vi "main2.vi"() -> ()   [LabVIEW 2015]
uses:
  myControl/calculationButton.ctl
  myControl/ChoseFromGraph.ctl
  myControl/Ok.ctl
  myControl/stopButton.ctl
  myControl/Events.ctl
  myControl/State.ctl
  <vilib>/Analysis/baseanly.llb/Mean (DBL).vi
  <vilib>/measure/mamon.llb/Waveform Peak Detection for 1 Chan.vi
  <vilib>/measure/NI_MAPro.lvlib
  <vilib>/Analysis/NI_AALBase.lvlib
panel:
  out "Title":string="Oscillatory Breathing Detection (beta 1.3)"
  in  "File Index:":path
  in  "Width (s):":i32
  in  "Threshold (L/min):":dbl format="%#.2g"
  in  "Low Cut-off (Hz):":dbl
  in  "OK Button":T1
  in  "ChooseFromGraph":T2
  in  "Calculate":T3
  in  "Stop Button":bool
  out "Ventilation":cluster{"Y":dbl[], "Y":dbl[]}[](graph)=[{"Y"=array[6401 elements], "Y"=array[8192 elements]}, {"Y"=[2.0, 11.0, 13.0, 16.0, 17.0, 20.0, 22.0, 24.0, 27.0, 30.0, 32.0, 36.0, 37.0, 40.0, 43.0, 45.0, 48.0, 51.0, 53.0, 55.0, 57.0, 61.0, 64.0, 66.0, 68.0, 71.0, 73.0, 75.0, 78.0, 81.0, 84.0, 86.0, 89.0, 92.0, 93.0, 96.0, 99.0, 101.0, 103.0, 107.0, 109.0, 112.0, 115.0, 118.0, 120.0, 124.0, 127.0, 129.0, 132.0, 134.0, 138.0], "Y"=[10.8, 11.5, 6.4, 8.0, 9.0, 13.8, 11.9, 14.1, 11.5, 15.7, 10.1, 14.3, 19.8, 19.2, 16.5, 21.5, 18.1, 18.9, 16.0, 17.4, 14.8, 15.3, 12.8, 11.8, 11.0, 12.4, 11.2, 12.5, 12.3, 11.5, 21.7, 21.2, 19.1, 23.7, 21.3, 20.4, 21.9, 18.3, 18.8, 17.7, 12.9, 12.6, 11.4, 9.9, 11.1, 12.3, 15.6, 14.5, 16.0, 14.2, 16.4]}]
  out "Duration (s)":dbl[](array[numeric]) format="%#.2g"
  out "Amplitude (L/min)":dbl[](array[numeric]) format="%#.2g"
  out "Mean Area Ratio":dbl format="%#.2g"
  out "Mean Area":dbl format="%#.2f"
  out "iValesLocation(samples)":dbl[](array[numeric])=[127.0, 3160.0, 5625.0] format="%#.2g"
  out "Cycle Number":i32
  out "EOB Ratio":dbl format="%#.2g"
  out "Freq. (1/min)":dbl format="%#.2g"
  out "Ampl. (L/min)":dbl format="%#.2g"
  out "DataArray":T4
  out "State Bar":string="Set the Run-Time settings and press Calculate Button "
  # "Preliminary Setting:"
  # "Run-Time Setting:"
  # "Detected cycles:"
  # "Average values:"
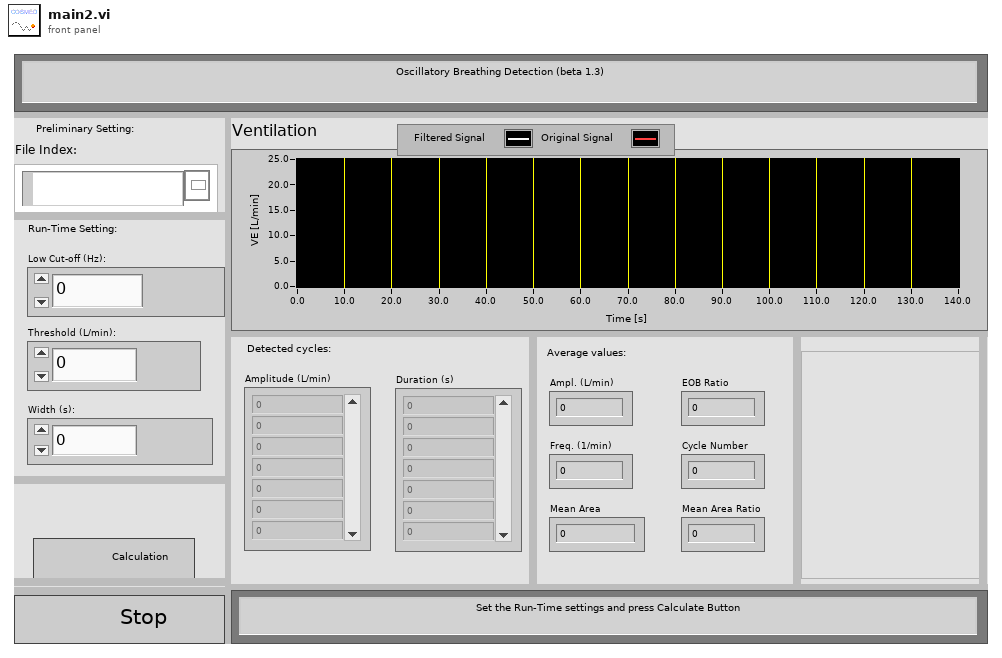
[diagram p1: front panel]
types:
  T1 = typedef "Ok.ctl" = bool
  T2 = typedef "ChoseFromGraph.ctl" = bool
  T3 = typedef "calculationButton.ctl" = bool
  T4 = cluster{"VE_E":dbl[], "time_E":dbl[], "VE_B":dbl[], "time_B":dbl[], "VE_E_noInter":dbl[], "time_E_noInter":dbl[], "VE_B_noInter":dbl[], "time_B_noInter":dbl[], "filteredSignal":dbl[], "iPeaksLocation":dbl[], "peaksAmplitude":dbl[], "valesAmplitude":dbl[], "iValesLocation":dbl[], "#_peaksFound":i32, "iPeakLocation_User":dbl[], "peakAmplitude_User":dbl[]}
  T5 = typedef "stopButton.ctl" = bool
  T6 = typedef "State.ctl" = enum16{"Inizializing", "UpLoad&ControlFile", "CalculationDefaultWidth", "WaitEvent", "Filter", "ChooseFromGraph", "FindPeaks", "FindVales", "TestOscillation", "CalculationOscillation", "Stop"}
  T7 = typedef "Events.ctl" = enum16{"WaitEvent", "ChoseFile", "Calculate", "ChoseFromGraoph", "Stop"}
  T8 = cluster{"time_E_noInter":dbl[], "VE_E_noInter":dbl[]}
  T9 = cluster{"time_E_noInter":dbl[], "VE_E_noInter":dbl[]}[]
  T10 = typedef "LVPoint32TypeDef.ctl" = cluster{"Horizontal":i32, "Vertical":i32}
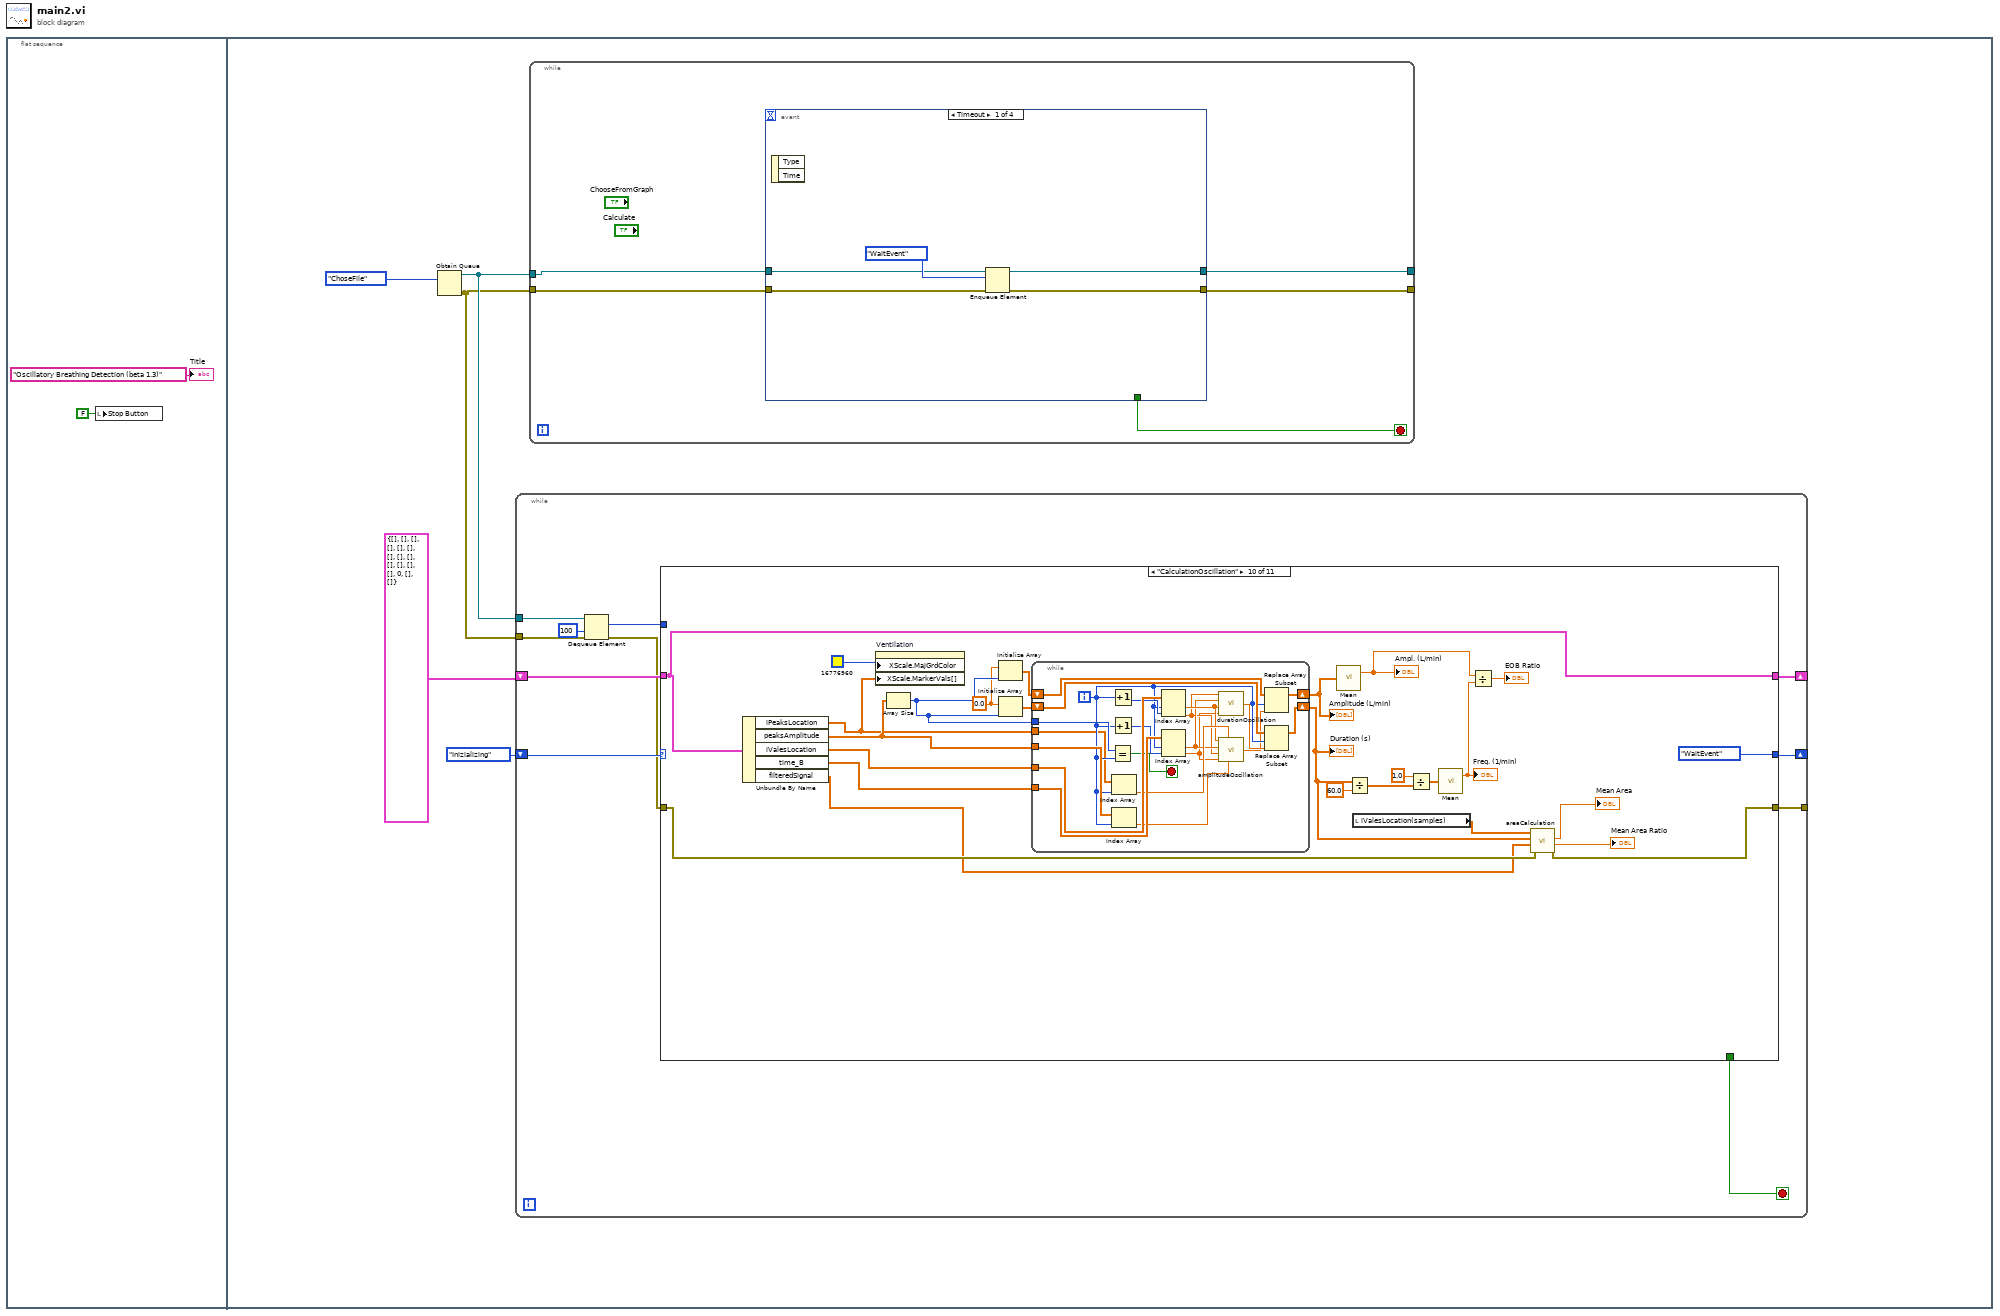
[diagram p0: block diagram]
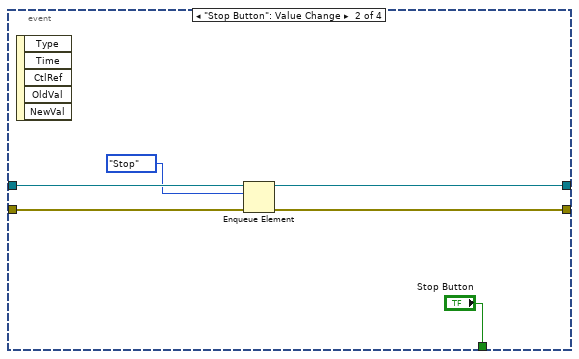
[diagram p2: hidden frame]
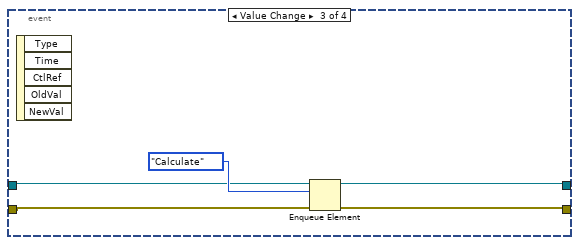
[diagram p3: hidden frame]
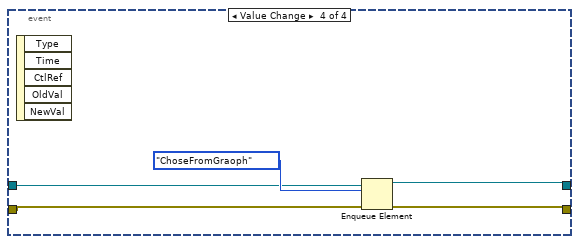
[diagram p4: hidden frame]
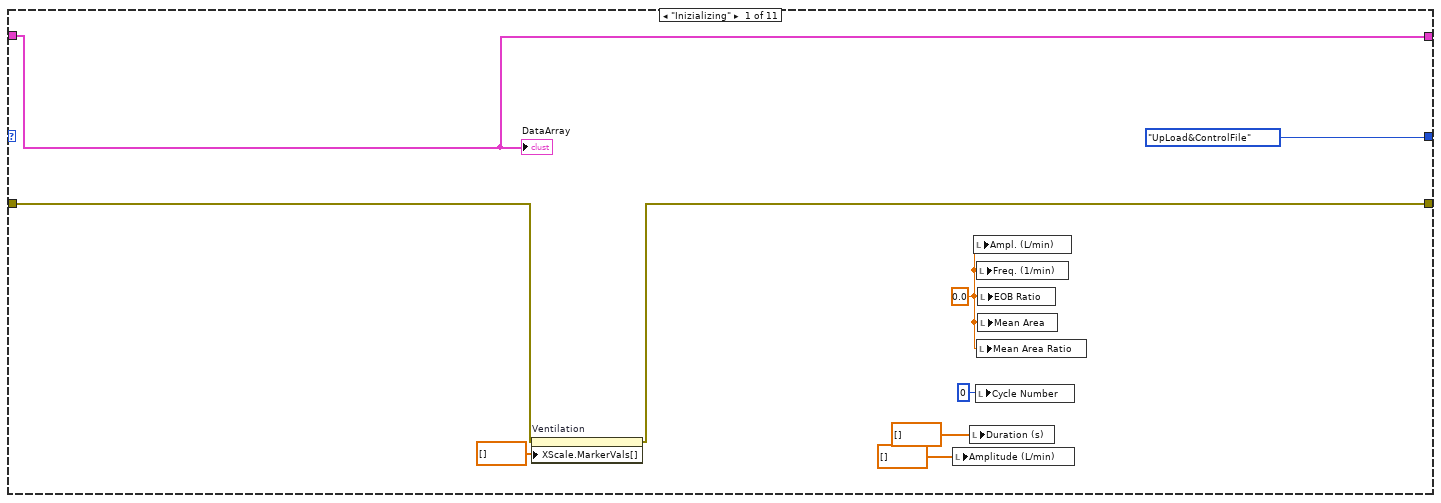
[diagram p5: hidden frame]
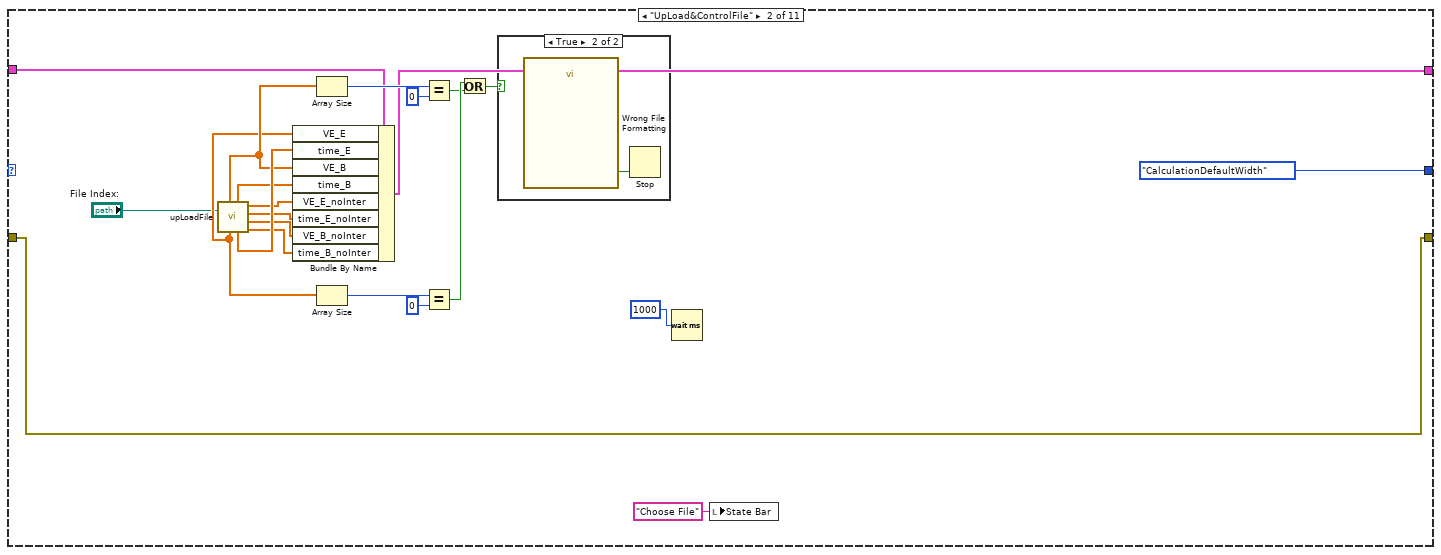
[diagram p6: hidden frame]
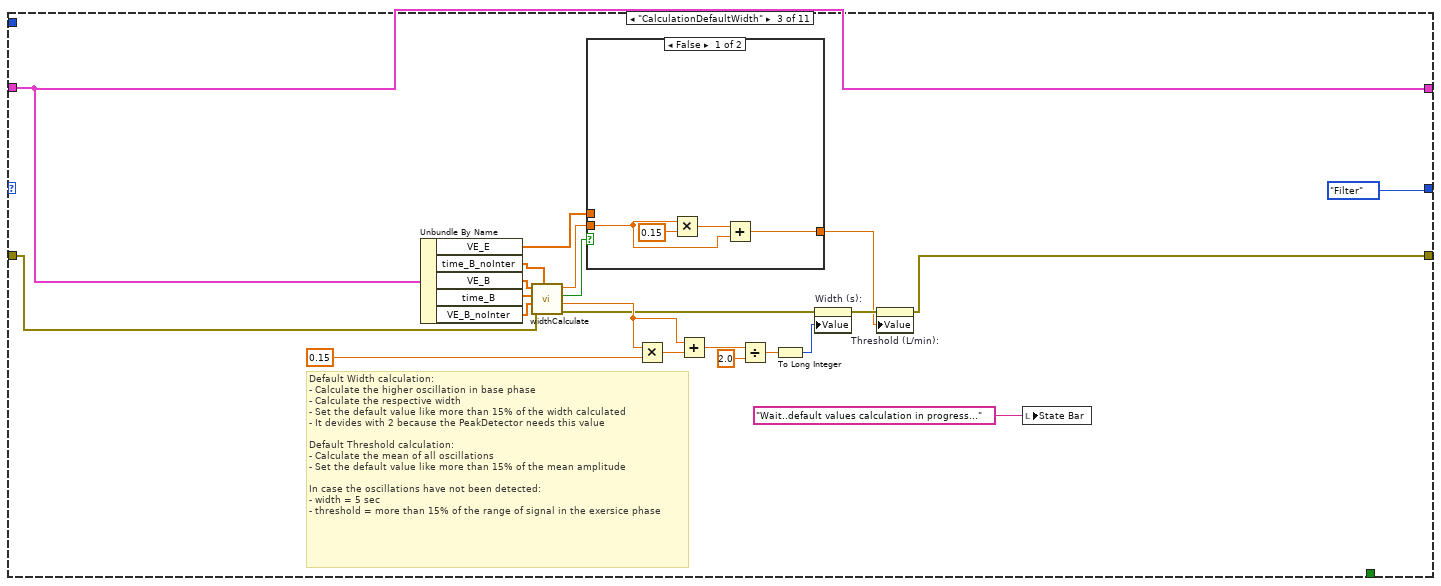
[diagram p8: hidden frame]
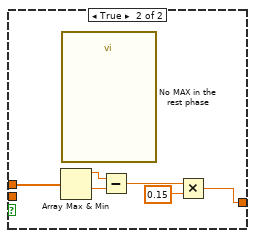
[diagram p9: hidden frame]
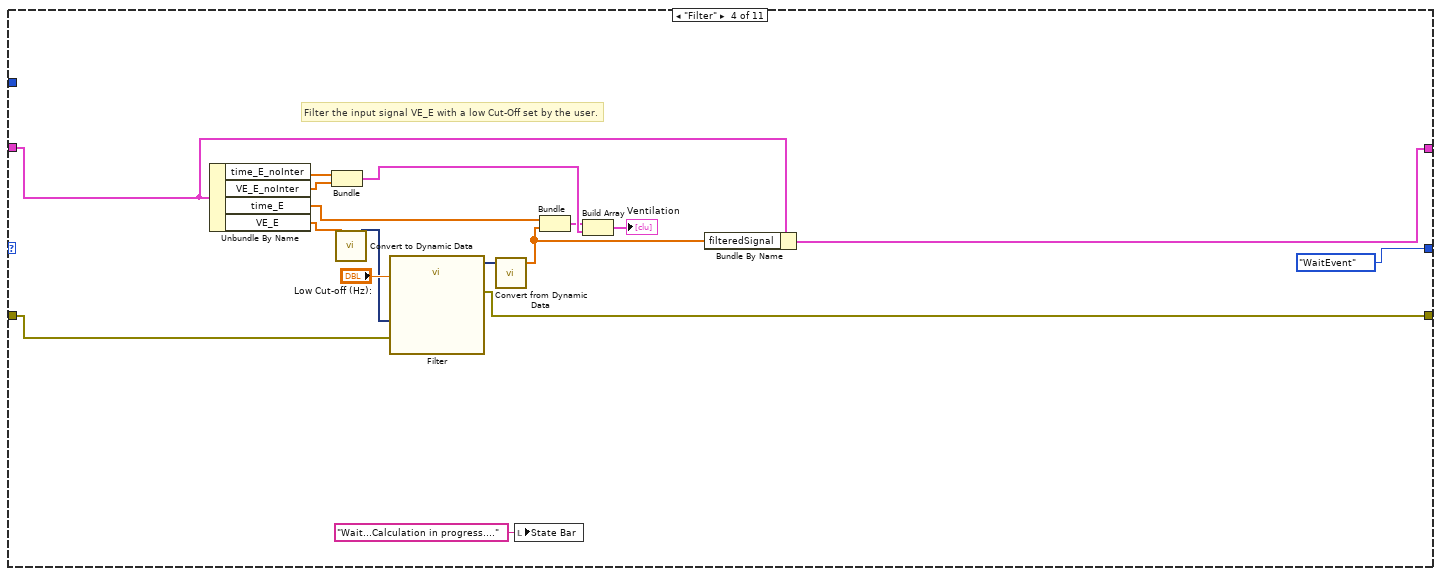
[diagram p10: hidden frame]
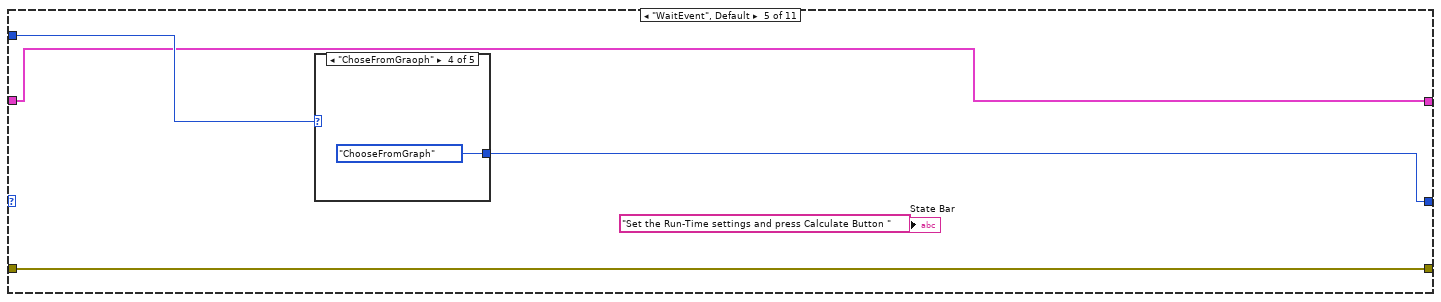
[diagram p11: hidden frame]
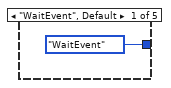
[diagram p12: hidden frame]
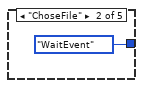
[diagram p13: hidden frame]
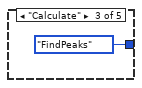
[diagram p14: hidden frame]
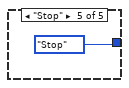
[diagram p15: hidden frame]
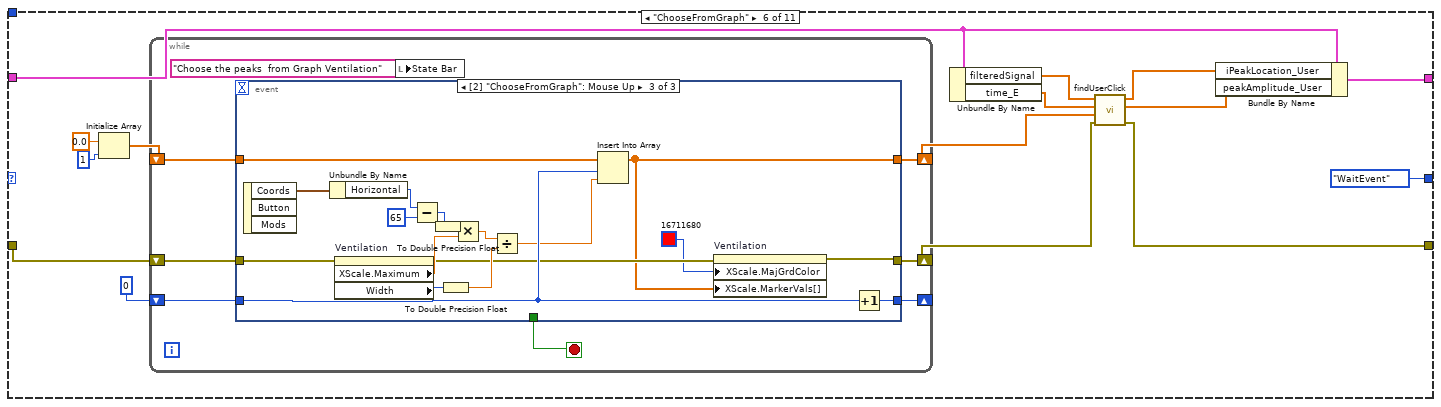
[diagram p16: hidden frame]
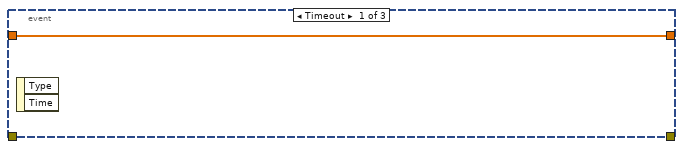
[diagram p17: hidden frame]
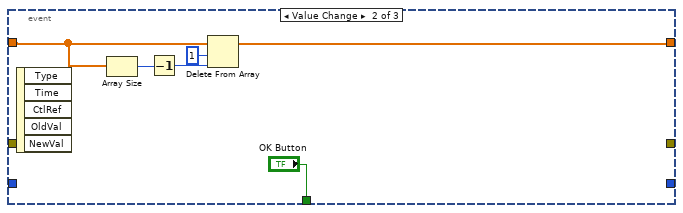
[diagram p18: hidden frame]
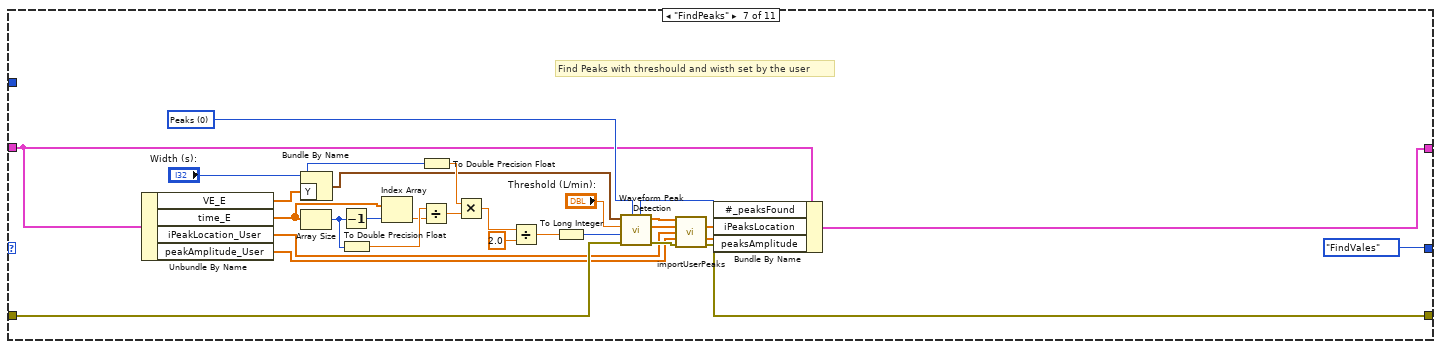
[diagram p19: hidden frame]
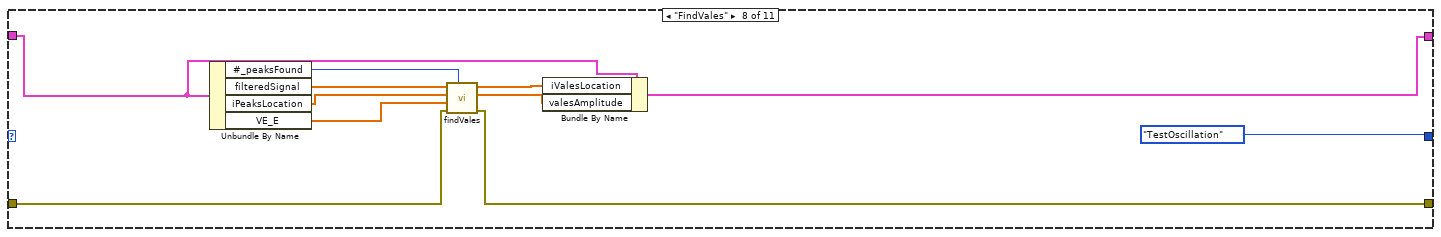
[diagram p20: hidden frame]
diagram:
  n1 = flat-sequence {
    frame #0 {
      n2 = local write "Stop Button"(T5 FALSE ("Stop Button")) -> ()
      "Title" <- "Oscillatory Breathing Detection (beta 1.3)" ("String")
    }
    frame #1 {
      n3 = Obtain Queue(element data type=Events."ChoseFile" ("Events")) -> (queue out=w7:refnum<queue>, error out=w6:errorcluster)  [unwired: 4 in, 1 out]
      n4 = while {
        shift-right: [w43] -> _
        shift-left: State."Inizializing" ("States") -> [w44]
        tunnel: w7 -> [w42]
        tunnel: w6 -> [w41]
        shift-right: [w39] -> _
        shift-left: T4 {"VE_E"=[], "time_E"=[], "VE_B"=[], "time_B"=[], "VE_E_noInter"=[], "time_E_noInter"=[], "VE_B_noInter"=[], "time_B_noInter"=[], "filteredSignal"=[], "iPeaksLocation"=[], "peaksAmplitude"=[], "valesAmplitude"=[], "iValesLocation"=[], "#_peaksFound"=0, "iPeakLocation_User"=[], "peakAmplitude_User"=[]} ("DataArray 2") -> [w38]
        tunnel: [w36] -> _
        stop <- w34 stop-if-true
        n5 = Dequeue Element(queue=w42, timeout in ms (-1)=100, error in (no error)=w41) -> (element=w35:T7, error out=w37:errorcluster)  [unwired: 2 out]
        n6 = case shown="\"CalculationOscillation\"" w44 {
          tunnel: [State."UpLoad&ControlFile" ("States") State."CalculationDefaultWidth" ("States") State."Filter" ("States") State."WaitEvent" ("States") w129 State."WaitEvent" ("States") State."FindVales" ("States") State."TestOscillation" ("States") State."CalculationOscillation" ("States") State."WaitEvent" ("States") State."WaitEvent" ("States")] -> w43
          tunnel: w38 -> [w52 w58 w83 w113 w128 w143 w196 w217 w238 w284 w324]
          tunnel: [w52 w56 w83 w112 w128 w144 w195 w214 w237 w284 w324] -> w39
          tunnel: w37 -> [w50 w54 w85 w115 w127 w149 w194 w223 w250 w280 w321]
          tunnel: [w49 w54 w80 w114 w127 w141 w190 w222 w240 w279 w321] -> w36
          tunnel: w35 -> [_ _ _ _ w130 _ _ _ _ _ _]
          tunnel: [_ _ _ _ _ _ _ _ _ _ TRUE] -> w34
          frame "Inizializing" {
            w45 = 0.0 ("Ampl. (L/min)")
            n7 = property on="Ventilation" class="XYGraph (strict)"(error in=w50, "XScale.MarkerVals[]"=dbl[] [] ("X Scale.Marker Values[]")) -> (error out=w49:errorcluster)  [unwired: 1 in, 1 out]
            n8 = local write "Amplitude (L/min)"(dbl[] [] ("Amplitude (L/min)")) -> ()
            n9 = local write "Duration (s)"(dbl[] [] ("Duration (s)")) -> ()
            n10 = local write "Ampl. (L/min)"(w45) -> ()
            n11 = local write "Cycle Number"(0 ("Cycle Number")) -> ()
            n12 = local write "Freq. (1/min)"(w45) -> ()
            n13 = local write "Mean Area Ratio"(w45) -> ()
            n14 = local write "EOB Ratio"(w45) -> ()
            n15 = local write "Mean Area"(w45) -> ()
            "DataArray" <- w52
          }
          frame "UpLoad&ControlFile" {
            n16 = call "upLoadFile.vi"("file path (dialog if empty)"="File Index:") -> ("time_B_noInter"=w60:dbl[], "VE_B_noInter"=w61:dbl[], "time_E_noInter"=w62:dbl[], "VE_E_noInter"=w63:dbl[], "time_E"=w66:dbl[], "time_B"=w64:dbl[], "VE_E"=w59:dbl[], "VE_B"=w65:dbl[])  [unwired: 3 in]
            n17 = Bundle By Name(cluster=w58, "VE_E"=w59, "time_E"=w66, "VE_B"=w65, "time_B"=w64, "VE_E_noInter"=w63, "time_E_noInter"=w62, "VE_B_noInter"=w61, "time_B_noInter"=w60) -> (w56:T4)
            n18 = Array Size(array=w65) -> (size(s)=w69:i32)
            n19 = Array Size(array=w59) -> (size(s)=w73:i32)
            n20 = Equal?(x=w69, y=0) -> (x = y?=w67:bool)
            n21 = Equal?(x=w73, y=0) -> (x = y?=w71:bool)
            n22 = Or(x=w71, y=w67) -> (x .or. y?=w70:bool)
            n23 = case shown="True" w70 {
              frame False {
              }
              frame True {
                n24 = call "Wrong File Formatting"() -> ("OK"=w76:bool)  [unwired: 10 in, 1 out]
                n25 = Stop(stop? (T)=w76) -> ()
              }
            }
            n26 = Wait (ms)(milliseconds to wait=u32 1000) -> ()  [unwired: 1 out]
            n27 = local write "State Bar"("Choose File" ("State Bar")) -> ()
          }
          frame "CalculationDefaultWidth" {
            # "Default Width calculation:\n- Calculate the higher oscillation in base phase\n- Calculate the respective width\n- Set the default value like more than 15% of the width calculated\n- It devides with 2 because the PeakDetector needs this value\n\nDefault Threshold calculation:\n- Calculate the mean of all oscillations\n- Set the default value like more than 15% of the mean amplitude\n\nIn case the oscillations have not been detected:\n- width = 5 sec\n- threshold = more than 15% of the range of signal in the exersice phase"
            n28 = Unbundle By Name(w83) -> ("VE_E"=w77:dbl[], "time_B_noInter"=w86:dbl[], "VE_B"=w89:dbl[], "time_B"=w88:dbl[], "VE_B_noInter"=w87:dbl[])
            n29 = call "widthCalculate.vi"("time_B_noInter"=w86, "Error In"=w85, "VE_B_noInter"=w87, "time_B"=w88, "VE_B"=w89) -> ("Error Out"=w82:errorcluster, "maxWidth"=w93:dbl, "noMin"=w98:bool, "Ampl. (L/min)"=w79:dbl)
            n30 = case shown="False" w98 {
              tunnel: w79 -> [w100 _]
              tunnel: [w99 w103] -> w78
              tunnel: w77 -> [_ w108]
              frame False {
                n31 = Multiply(x=w100, y=0.15) -> (x*y=w101:dbl)
                n32 = Add(x=w101, y=w100) -> (x+y=w99:dbl)
              }
              frame True {
                n33 = Array Max & Min(array=w108) -> (max value=w107:dbl, min value=w106:dbl)  [unwired: 2 out]
                n34 = call "No MAX in the rest phase"() -> ()  [unwired: 10 in, 2 out]
                n35 = Subtract(x=w107, y=w106) -> (x-y=w105:dbl)
                n36 = Multiply(x=w105, y=0.15) -> (x*y=w103:dbl)
              }
            }
            n37 = Multiply(x=w93, y=0.15) -> (x*y=w92:dbl)
            n38 = Add(x=w93, y=w92) -> (x+y=w91:dbl)
            n39 = Divide(x=w91, y=2.0) -> (x/y=w95:dbl)
            n40 = To Long Integer(number=w95) -> (32bit integer=w90:i32)
            n41 = property on="Width (s):" class="DigNum (strict)"(error in=w82, "Value"=w90) -> (error out=w81:errorcluster)  [unwired: 1 in, 1 out]
            n42 = property on="Threshold (L/min):" class="DigNum (strict)"(error in=w81, "Value"=w78) -> (error out=w80:errorcluster)  [unwired: 1 in, 1 out]
            n43 = local write "State Bar"("Wait..default values calculation in progress..." ("State Bar")) -> ()
          }
          frame "Filter" {
            # "Filter the input signal VE_E with a low Cut-Off set by the user."
            n44 = Unbundle By Name(w113) -> ("time_E_noInter"=w119:dbl[], "VE_E_noInter"=w118:dbl[], "time_E"=w117:dbl[], "VE_E"=w116:dbl[])
            n45 = Bundle("time_E_noInter"=w119, "VE_E_noInter"=w118) -> (w125:T8)  [unwired: 1 in]
            n46 = call "Convert to Dynamic Data"("Array"=w116) -> ("Dynamic Data Type"=w121:dynamicdata)  [unwired: 3 in]
            n47 = call "Filter"("error in (no error)"=w115, "Lower Cut-Off"="Low Cut-off (Hz):", "Signal"=w121) -> ("error out"=w114:errorcluster, "Filtered Signal"=w122:dynamicdata)  [unwired: 7 in]
            n48 = call "Convert from Dynamic Data"("Dynamic Data Type"=w122) -> ("Array"=w109:dbl[])  [unwired: 3 in]
            n49 = local write "State Bar"("Wait...Calculation in progress...." ("String 2")) -> ()
            n50 = Bundle("time_E"=w117, "Array"=w109) -> (w123:cluster{"time_E":dbl[], "Array":dbl[]})  [unwired: 1 in]
            n51 = Build Array(w123, w125) -> (→"Ventilation":T9)
            n52 = Bundle By Name(cluster=w113, "filteredSignal"=w109) -> (w112:T4)
          }
          frame "WaitEvent", Default {
            n53 = case shown="\"ChoseFromGraoph\"" w130 {
              tunnel: [State."WaitEvent" ("States") State."WaitEvent" ("States") State."FindPeaks" ("States") State."ChooseFromGraph" ("States") State."Stop" ("States")] -> w129
              frame "WaitEvent", Default {
              }
              frame "ChoseFile" {
              }
              frame "Calculate" {
              }
              frame "ChoseFromGraoph" {
              }
              frame "Stop" {
              }
            }
            "State Bar" <- "Set the Run-Time settings and press Calculate Button " ("State Bar")
          }
          frame "ChooseFromGraph" {
            n54 = Initialize Array(0.0 ("element"), 1 ("dimension size")) -> (w145:dbl[])
            n55 = while {
              shift-right: [w152] -> w142
              shift-left: w149 -> [w158]
              shift-right: [w154] -> w140
              shift-left: w145 -> [w157]
              shift-right: [w155] -> _
              shift-left: 0 ("element") -> [w156]
              stop <- w151 stop-if-true
              n56 = event shown="[2] \"ChooseFromGraph\": Mouse Up" {
                selector: _ -> [_ _ _]
                dyn-events: _ -> [_ _ _]
                timeout: _ -> [_ _ _]
                tunnel: w158 -> [_ _ w183]
                tunnel: w157 -> [w159 w164 w172]
                tunnel: w156 -> [_ _ w171]
                tunnel: [_ _ w173] -> w155
                tunnel: [w159 w165 w167] -> w154
                tunnel: [_ _ w168] -> w152
                tunnel: [_ "OK Button" _] -> w151
                event Timeout {
                  n57 = event-data() -> ()  [unwired: 1 in, 2 out]
                }
                event Value Change {
                  n58 = event-data() -> ()  [unwired: 1 in, 5 out]
                  n59 = Array Size(array=w164) -> (size(s)=w163:i32)
                  n60 = Decrement(x=w163) -> (x-1=w161:i32)
                  n61 = Delete From Array(array=w164, length=1, index=w161) -> (array with subset deleted=w165:dbl[])  [unwired: 1 out]
                }
                event Mouse Up {
                  n62 = event-data() -> ("Coords"=w182:T10)  [unwired: 1 in, 2 out]
                  n63 = Unbundle By Name(w182) -> ("Horizontal"=w181:i32)
                  n64 = property on="Ventilation" class="XYGraph (strict)"(error in=w183) -> (error out=w169:errorcluster, "XScale.Maximum"=w179:dbl, "Width"=w175:u32)  [unwired: 1 in, 1 out]
                  n65 = Subtract(x=w181, y=65) -> (x-y=w178:i32)
                  n66 = To Double Precision Float(number=w178) -> (double precision float=w177:dbl)
                  n67 = To Double Precision Float(number=w175) -> (double precision float=w174:dbl)
                  n68 = Multiply(x=w177, y=w179) -> (x*y=w176:dbl)
                  n69 = Divide(x=w176, y=w174) -> (x/y=w170:dbl)
                  n70 = Insert Into Array(array=w172, index=w171, new element=w170) -> (w167:dbl[])
                  n71 = property on="Ventilation" class="XYGraph (strict)"(error in=w169, "XScale.MajGrdColor"=u32 16711680 ("Color Box"), "XScale.MarkerVals[]"=w167) -> (error out=w168:errorcluster)  [unwired: 1 in, 1 out]
                  n72 = Increment(x=w171) -> (x+1=w173:i32)
                }
              }
              n73 = local write "State Bar"("Choose the peaks  from Graph Ventilation" ("State Bar")) -> ()
            }
            n74 = Unbundle By Name(w143) -> ("filteredSignal"=w138:dbl[], "time_E"=w139:dbl[])
            n75 = call "findUserClick.vi"("Error In"=w142, "clickLocation"=w140, "time_E"=w139, "VE_amplitude"=w138) -> ("Error Out"=w141:errorcluster, "amplitudePeaks"=w136:dbl[], "iPeaksLocation"=w137:dbl[])  [unwired: 5 in]
            n76 = Bundle By Name(cluster=w143, "iPeakLocation_User"=w137, "peakAmplitude_User"=w136) -> (w144:T4)
          }
          frame "FindPeaks" {
            w200 = u16 0 items=["Peaks", "Valleys"] ("peaks/valleys")
            # "Find Peaks with threshould and wisth set by the user"
            n77 = Unbundle By Name(w196) -> ("VE_E"=w197:dbl[], "time_E"=w198:dbl[], "iPeakLocation_User"=w185:dbl[], "peakAmplitude_User"=w184:dbl[])
            n78 = Bundle By Name("Y"=w197) -> (w201:waveform(dbl))  [unwired: 1 in]
            n79 = Array Size(array=w198) -> (size(s)=w209:i32)
            n80 = Decrement(x=w209) -> (x-1=w211:i32)
            n81 = To Double Precision Float(number=w209) -> (double precision float=w210:dbl)
            n82 = Index Array(array=w198, index=w211) -> (element=w199:dbl)
            n83 = Divide(x=w210, y=w199) -> (x/y=w212:dbl)
            n84 = To Double Precision Float(number="Width (s):") -> (double precision float=w204:dbl)
            n85 = Multiply(x=w204, y=w212) -> (x*y=w206:dbl)
            n86 = Divide(x=w206, y=2.0) -> (x/y=w208:dbl)
            n87 = To Long Integer(number=w208) -> (32bit integer=w205:i32)
            n88 = call-poly <vilib>:"Waveform Peak Detection.vi"("peaks/valleys"=w200, "error in"=w194, "width"=w205, "threshold"="Threshold (L/min):", "Signal In"=w201) -> ("error out"=w191:errorcluster, "Amplitudes"=w187:dbl[], "Locations"=w186:dbl[], "# found"=w193:i32)  [unwired: 2 in, 1 out]
            n89 = call "importUserPeaks.vi"("iPeak_Location"=w186, "amplitudePeaks"=w187, "iPeak_LocationUSER"=w185, "amplitudePeaksUSER"=w184, "Error In"=w191) -> ("iPeak_LocationFinal"=w189:dbl[], "amplitudePeaksFinal"=w188:dbl[], "Error Out"=w190:errorcluster)  [unwired: 8 in]
            n90 = Bundle By Name(cluster=w196, "#_peaksFound"=w193, "iPeaksLocation"=w189, "peaksAmplitude"=w188) -> (w195:T4)
          }
          frame "FindVales" {
            n91 = Unbundle By Name(w217) -> ("#_peaksFound"=w221:i32, "filteredSignal"=w220:dbl[], "iPeaksLocation"=w219:dbl[], "VE_E"=w218:dbl[])
            n92 = call "findVales.vi"("#_foundPeaks"=w221, "Error In"=w223, "VE_E"=w218, "iPeaksLocation"=w219, "filteredSignal"=w220) -> ("Error Out"=w222:errorcluster, "valesAmplitude"=w215:dbl[], "iValesLocation"=w216:dbl[])  [unwired: 4 in]
            n93 = Bundle By Name(cluster=w217, "iValesLocation"=w216, "valesAmplitude"=w215) -> (w214:T4)
          }
          frame "TestOscillation" {
            w245 = 0.0 ("element")
            n94 = local read "Threshold (L/min):"() -> (w251:dbl)
            n95 = Unbundle By Name(w238) -> ("#_peaksFound"=w254:i32, "valesAmplitude"=w253:dbl[], "peaksAmplitude"=w252:dbl[])
            n96 = Unbundle By Name(w238) -> ("time_E"=w239:dbl[], "filteredSignal"=w231:dbl[], "peaksAmplitude"=w230:dbl[], "iValesLocation"=w225:dbl[], "iPeaksLocation"=w229:dbl[], "valesAmplitude"=w228:dbl[])
            n97 = call "verifyThreshold.vi"("#Peaks"=w254, "valesAmplitude"=w253, "peaksAmplitude"=w252, "Error In"=w250, "threshold"=w251) -> ("passThreshold"=w249:i32[], "Error Out"=w248:errorcluster)
            n98 = call "testMaxMin.vi"("valesAmplitude in"=w228, "peaksAmplitude in"=w230, "Error In"=w248, "iPeaksLocation in"=w229, "iValesLocation in"=w225, "passThreshold"=w249) -> ("Error Out"=w242:errorcluster, "iValesLocation out"=w224:dbl[], "valesAmplitude out"=w233:dbl[])  [unwired: 2 out]
            "iValesLocation(samples)" <- w224
            n99 = Array Size(array=w224) -> (size(s)=w227:i32)
            n100 = call "iToTime.vi"("Error In"=w242, "time"=w239, "iArray"=w224) -> ("Error Out"=w241:errorcluster, "timeArray"=w234:dbl[])
            n101 = Decrement(x=w227) -> (x-1=w226:i32)
            "Cycle Number" <- w226
            n102 = Initialize Array(w245, w226) -> (w244:dbl[])
            n103 = Initialize Array(w245, w226) -> (w246:dbl[])
            n104 = while {
              tunnel: w224 -> [w273]
              tunnel: w227 -> [w272]
              tunnel: w231 -> [w269]
              shift-right: [w255] -> _
              shift-left: 0 -> [w256]
              shift-right: [w266] -> w235
              shift-left: w246 -> [w267]
              shift-right: [w264] -> w243
              shift-left: w244 -> [w265]
              i -> [w263]
              stop <- w271 stop-if-true
              n105 = Increment(x=w263) -> (x+1=w259:i32)
              n106 = Equal?(x=w272, y=w263) -> (x = y?=w271:bool)
              n107 = Index Array(array=w273, index=w259) -> (element=w270:dbl)
              n108 = To Long Integer(number=w270) -> (32bit integer=w255:i32)
              n109 = Subtract(x=w255, y=w256) -> (x-y=w257:i32)
              n110 = Array Subset(array=w269, index=w256, length=w257) -> (w268:dbl[])
              n111 = Array Max & Min(array=w268) -> (max value=w261:dbl, max index (indices)=w262:i32)  [unwired: 2 out]
              n112 = Add(x=w262, y=w256) -> (x+y=w258:i32)
              n113 = Replace Array Subset(array=w267, new element=w261, index=w263) -> (w266:dbl[])
              n114 = To Double Precision Float(number=w258) -> (double precision float=w260:dbl)
              n115 = Replace Array Subset(array=w265, new element=w260, index=w263) -> (w264:dbl[])
            }
            n116 = call "iToTime.vi"("Error In"=w241, "time"=w239, "iArray"=w243) -> ("Error Out"=w240:errorcluster, "timeArray"=w236:dbl[])
            n117 = Bundle By Name(cluster=w238, "valesAmplitude"=w233, "iPeaksLocation"=w236, "peaksAmplitude"=w235, "iValesLocation"=w234) -> (w237:T4)
          }
          frame "CalculationOscillation" {
            w288 = 0.0 ("element")
            n118 = Unbundle By Name(w284) -> ("iPeaksLocation"=w282:dbl[], "peaksAmplitude"=w287:dbl[], "iValesLocation"=w286:dbl[], "time_B"=w285:dbl[], "filteredSignal"=w276:dbl[])
            n119 = property on="Ventilation" class="XYGraph (strict)"("XScale.MajGrdColor"=u32 16776960 ("Color Box"), "XScale.MarkerVals[]"=w282) -> ()  [unwired: 2 in, 2 out]
            n120 = Array Size(array=w287) -> (size(s)=w299:i32)
            n121 = Initialize Array(w288, w299) -> (w289:dbl[])
            n122 = Initialize Array(w288, w299) -> (w290:dbl[])
            n123 = while {
              tunnel: w287 -> [w320]
              tunnel: w282 -> [w300]
              tunnel: w285 -> [w319]
              tunnel: w286 -> [w318]
              tunnel: w299 -> [w317]
              shift-right: [w310] -> w277
              shift-left: w290 -> [w311]
              shift-right: [w312] -> w291
              shift-left: w289 -> [w313]
              i -> [w309]
              stop <- w316 stop-if-true
              n124 = Equal?(x=w317, y=w309) -> (x = y?=w316:bool)
              n125 = Increment(x=w309) -> (x+1=w314:i32)
              n126 = Increment(x=w309) -> (x+1=w315:i32)
              n127 = Index Array(array=w300, index=w309) -> (element=w307:dbl)
              n128 = Index Array(array=w320, index=w309) -> (element=w306:dbl)
              n129 = Index Array(array=w318, index #1=w309, index #2=w314) -> (element #1=w305:dbl, element #2=w303:dbl)
              n130 = Index Array(array=w319, index #1=w309, index #2=w315) -> (element #1=w304:dbl, element #2=w302:dbl)
              n131 = call "durationOscillation.vi"("valesAmplitude2"=w302, "timeValesLocation1"=w305, "valesAmplitude1"=w304, "timeValesLocation2"=w303) -> ("durationOscilation"=w308:dbl)
              n132 = call "amplitudeOscillation.vi"("y0"=w306, "x0"=w307, "y2"=w302, "x2"=w303, "y1"=w304, "x1"=w305) -> ("amplitudeOscillation"=w301:dbl)
              n133 = Replace Array Subset(array=w313, new element=w301, index=w309) -> (w312:dbl[])
              n134 = Replace Array Subset(array=w311, new element=w308, index=w309) -> (w310:dbl[])
            }
            "Duration (s)" <- w277
            "Amplitude (L/min)" <- w291
            n135 = call-poly <vilib>:"Mean.vi"("X"=w291) -> ("mean"=w295:dbl)  [unwired: 1 out]
            "Ampl. (L/min)" <- w295
            n136 = Divide(x=w277, y=60.0) -> (x/y=w293:dbl[])
            n137 = local read "iValesLocation(samples)"() -> (w278:dbl[])
            n138 = Divide(x=1.0, y=w293) -> (x/y=w297:dbl[])
            n139 = call-poly <vilib>:"Mean.vi"("X"=w297) -> ("mean"=w298:dbl)  [unwired: 1 out]
            "Freq. (1/min)" <- w298
            n140 = Divide(x=w295, y=w298) -> (x/y=→"EOB Ratio":dbl)
            n141 = call "areaCalculation.vi"("error in (no error)"=w280, "filteredSignal"=w276, "Duration"=w277, "iValesLocation(Samples)"=w278) -> ("error out"=w279:errorcluster, "meanArea/numOsci"=→"Mean Area Ratio":dbl, "meanArea"=→"Mean Area":dbl)  [unwired: 5 in]
          }
          frame "Stop" {
          }
        }
      }
      n142 = while {
        tunnel: w7 -> [w12]
        tunnel: w6 -> [w11]
        tunnel: [w10] -> _
        tunnel: [w9] -> _
        stop <- w8 stop-if-true
        n143 = event shown="[0] Timeout" {
          selector: _ -> [_ _ _ _]
          dyn-events: _ -> [_ _ _ _]
          timeout: _ -> [_ _ _ _]
          tunnel: w12 -> [w16 w23 w27 w32]
          tunnel: w11 -> [w15 w22 w26 w31]
          tunnel: [w14 w21 w25 w30] -> w10
          tunnel: [w13 w20 w24 w29] -> w9
          tunnel: [_ "Stop Button" _ _] -> w8
          event Timeout {
            n144 = event-data() -> ()  [unwired: 1 in, 2 out]
            n145 = Enqueue Element(queue=w16, element=Events."WaitEvent" ("Events"), error in (no error)=w15) -> (queue out=w14:refnum<queue>, error out=w13:errorcluster)  [unwired: 1 in, 1 out]
          }
          event "Stop Button": Value Change {
            n146 = event-data() -> ()  [unwired: 1 in, 5 out]
            n147 = Enqueue Element(queue=w23, element=Events."Stop" ("Events"), error in (no error)=w22) -> (queue out=w21:refnum<queue>, error out=w20:errorcluster)  [unwired: 1 in, 1 out]
          }
          event Value Change {
            n148 = event-data() -> ()  [unwired: 1 in, 5 out]
            n149 = Enqueue Element(queue=w27, element=Events."Calculate" ("Events"), error in (no error)=w26) -> (queue out=w25:refnum<queue>, error out=w24:errorcluster)  [unwired: 1 in, 1 out]
          }
          event Value Change {
            n150 = event-data() -> ()  [unwired: 1 in, 5 out]
            n151 = Enqueue Element(queue=w32, element=Events."ChoseFromGraoph" ("Events"), error in (no error)=w31) -> (queue out=w30:refnum<queue>, error out=w29:errorcluster)  [unwired: 1 in, 1 out]
          }
        }
      }
    }
  }
